vi "Snap.vi"(8 "error in (no error)":errorcluster, 11 "reference in":refnum<class "Camera_IMAQdx.lvclass">) -> (0 "error out":errorcluster, 2 "Image Out":T1, 3 "reference out":refnum<class "Camera_IMAQdx.lvclass">)   [LabVIEW 2017, in "Camera_IMAQdx.lvclass"]
doc: "Snaps a single image. Does not require Start and Stop Acquisition."
uses:
  Camera_IMAQdx.lvclass
  <vilib>/vision/Image Controls.llb/IMAQ Image.ctl
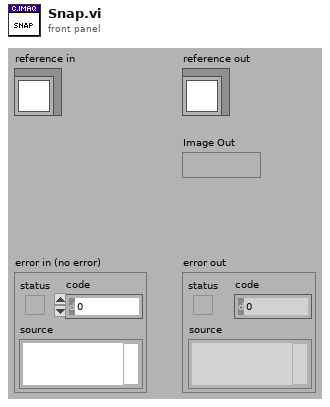
[diagram p1: front panel]
types:
  T1 = typedef "IMAQ Image.ctl" = refnum<image>
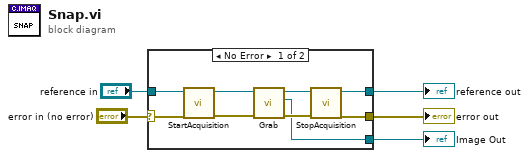
[diagram p0: block diagram]
diagram:
  n1 = case shown="No Error" "error in (no error)" {
    selector: "error in (no error)" -> [w8 w16]
    tunnel: [w7 w16] -> w4
    tunnel: [w11 w15] -> w2
    tunnel: "reference in" -> [w14 w15]
    tunnel: [w6 _] -> w1
    frame No Error {
      n2 = call-dynamic "StartAcquisition.vi"("error in (no error)"=w8, "reference in"=w14) -> ("error out"=w10:errorcluster, "reference out"=w13:refnum<class "Camera_IMAQdx.lvclass">)  [unwired: 8 in]
      n3 = call-dynamic "Grab.vi"("error in (no error)"=w10, "reference in"=w13) -> ("error out"=w9:errorcluster, "Image Out"=w6:T1, "reference out"=w12:refnum<class "Camera_IMAQdx.lvclass">)  [unwired: 6 in, 1 out]
      n4 = call-dynamic "StopAcquisition.vi"("error in (no error)"=w9, "reference in"=w12) -> ("error out"=w7:errorcluster, "reference out"=w11:refnum<class "Camera_IMAQdx.lvclass">)  [unwired: 8 in]
    }
    frame Error {
    }
  }
  "error out" <- w4
  "reference out" <- w2
  "Image Out" <- w1
